vi "BuildGRPCPackages.vi"(11 "CommandLineIn":string[](array[string])) -> (2 "output":string, 3 "return code":i32)   [LabVIEW 2019]
uses:
  <vilib>/JKI/VIPM API/VIPM API_vipm_api.lvlib
panel:
  # "* path to labview sources\n* labview version\n* labview bitness\n* Version"
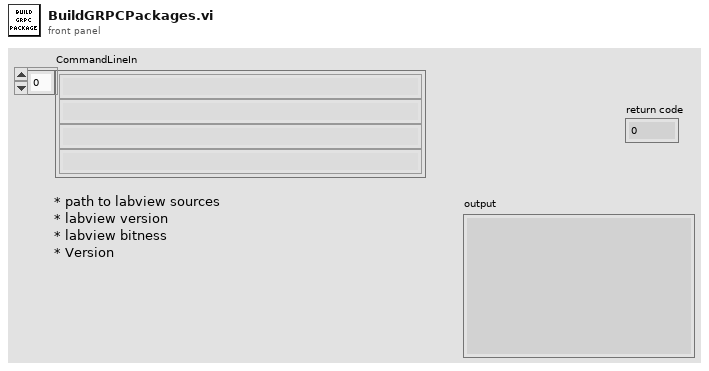
[diagram p1: front panel]
types:
  T1 = typedef "VIPM API_vipm_api.lvlib/LabVIEW Target Info Cluster_vipm_api.ctl" = cluster{"Version":string, "Connection Tested":bool, "Disabled":bool}
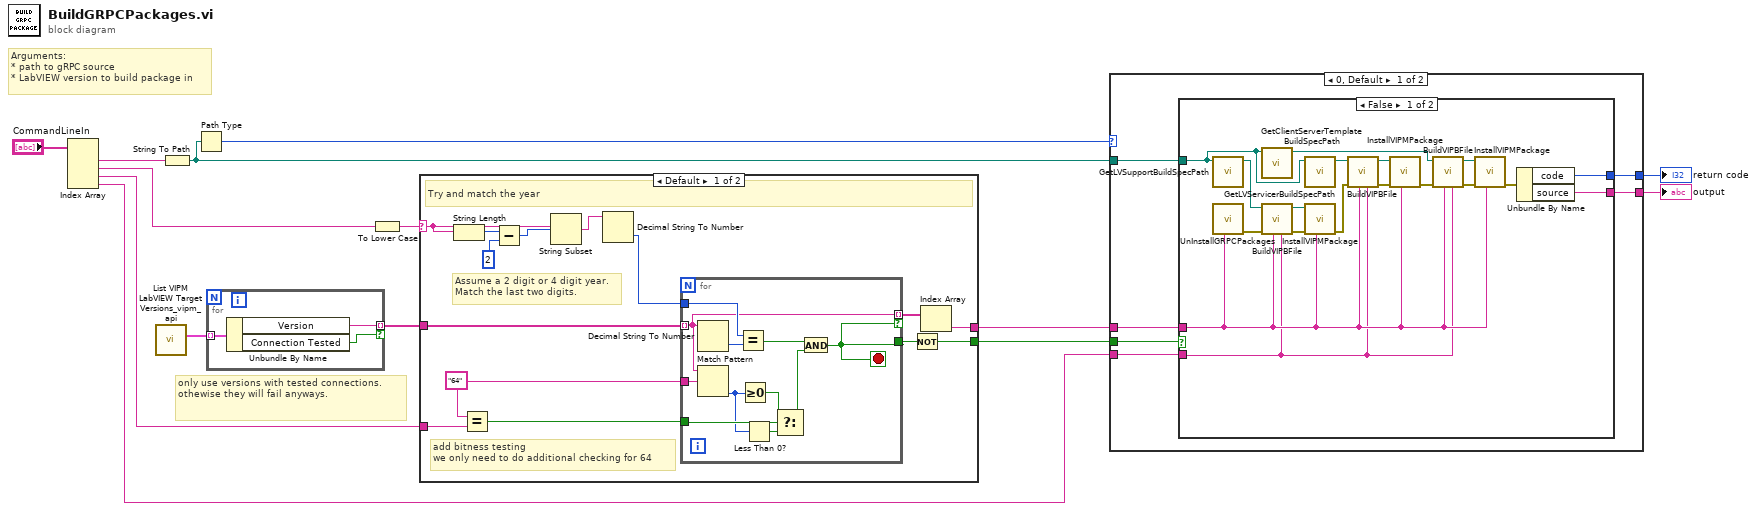
[diagram p0: block diagram]
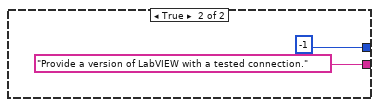
[diagram p2: hidden frame]
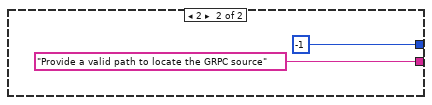
[diagram p3: hidden frame]
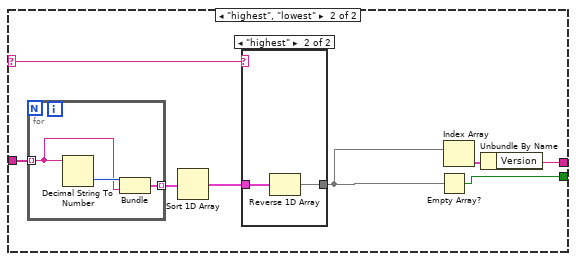
[diagram p4: hidden frame]
diagram:
  # "Arguments:\n* path to gRPC source\n* LabVIEW version to build package in"
  # "only use versions with tested connections.\nothewise they will fail anyways."
  n1 = Index Array(array="CommandLineIn") -> (element #1=w14:string, element #2=w5:string, element #3=w2:string, element #4=w1:string)  [unwired: 4 in]
  n2 = call <vilib>:"List VIPM LabVIEW Target Versions_vipm_api.vi"() -> ("LabVIEW Target Info"=w11:T1[])  [unwired: 10 in, 1 out]
  n3 = String To Path(string=w14) -> (path=w12:path)
  n4 = Path Type(1:w12) -> (0:w13:i16)
  n5 = for {
    tunnel: w11 -> [w17] mode=indexing
    tunnel: [w16] -> w9 mode=indexing if=w15
    n6 = Unbundle By Name(w17) -> ("Version"=w16:string, "Connection Tested"=w15:bool)
  }
  n7 = To Lower Case(string=w5) -> (all lower case string=w10:string)
  n8 = case shown="Default" w10 {
    selector: w10 -> [w31 w48]
    tunnel: w9 -> [w26 w50]
    tunnel: [w22 w45] -> w4
    tunnel: [w21 w43] -> w6
    tunnel: w2 -> [w20 _]
    frame Default {
      w18 = "64" ("x")
      # "add bitness testing\nwe only need to do additional checking for 64"
      # "Assume a 2 digit or 4 digit year.\nMatch the last two digits."
      # "Try and match the year"
      n9 = String Length(string=w31) -> (length=w30:i32)
      n10 = Equal?(x=w18, y=w20) -> (x = y?=w19:bool)
      n11 = Subtract(x=w30, y=2) -> (x-y=w28:i32)
      n12 = String Subset(string=w31, offset (0)=w28) -> (substring=w27:string)  [unwired: 1 in]
      n13 = Decimal String To Number(string=w27) -> (number=w25:i32)  [unwired: 2 in, 1 out]
      n14 = for {
        tunnel: w26 -> [w40] mode=indexing
        tunnel: w25 -> [w41]
        tunnel: [w34] -> w23
        tunnel: [w40] -> w24 mode=indexing if=w34
        tunnel: w19 -> [w37]
        tunnel: w18 -> [w39]
        stop <- w34 stop-if-true
        n15 = Decimal String To Number(string=w40) -> (number=w42:i32)  [unwired: 2 in, 1 out]
        n16 = Match Pattern(string=w40, regular expression=w39) -> (offset past match=w32:i32)  [unwired: 1 in, 3 out]
        n17 = Equal?(x=w41, y=w42) -> (x = y?=w36:bool)
        n18 = Greater Or Equal To 0?(x=w32) -> (x >= 0?=w38:bool)
        n19 = Less Than 0?(x=w32) -> (x < 0?=w33:bool)
        n20 = Select(t=w38, s=w37, f=w33) -> (s? t:f=w35:bool)
        n21 = And(x=w36, y=w35) -> (x .and. y?=w34:bool)
      }
      n22 = Not(x=w23) -> (.not. x?=w21:bool)
      n23 = Index Array(array=w24) -> (element=w22:string)  [unwired: 1 in]
    }
    frame "highest", "lowest" {
      n24 = for {
        tunnel: w50 -> [w55] mode=indexing
        tunnel: [w54] -> w49 mode=indexing
        n25 = Decimal String To Number(string=w55) -> (number=w56:i32)  [unwired: 2 in, 1 out]
        n26 = Bundle(w56, "Version"=w55) -> (w54:cluster{i32, "Version":string})  [unwired: 1 in]
      }
      n27 = Sort 1D Array(array=w49) -> (sorted array=w47:cluster{i32, "Version":string}[])
      n28 = case shown="\"highest\"" w48 {
        tunnel: w47 -> [w51 w53]
        tunnel: [w51 w52] -> w44
        frame Default {
        }
        frame "highest" {
          n29 = Reverse 1D Array(array=w53) -> (reversed array=w52:cluster{i32, "Version":string}[])
        }
      }
      n30 = Empty Array?(array=w44) -> (empty?=w43:bool)
      n31 = Index Array(array=w44) -> (element=w46:cluster{i32, "Version":string})  [unwired: 1 in]
      n32 = Unbundle By Name(w46) -> ("Version"=w45:string)
    }
  }
  n33 = case shown="0, Default" w13 {
    tunnel: [w60 -1 ("return code")] -> w8
    tunnel: [w61 "Provide a valid path to locate the GRPC source" ("Output")] -> w7
    tunnel: w12 -> [w62 _]
    tunnel: w6 -> [w59 _]
    tunnel: w4 -> [w58 _]
    tunnel: w1 -> [w57 _]
    frame 0, Default {
      n34 = case shown="False" w59 {
        tunnel: w62 -> [w78 _]
        tunnel: [w77 "Provide a version of LabVIEW with a tested connection." ("Output")] -> w61
        tunnel: [w76 -1 ("return code")] -> w60
        tunnel: w58 -> [w64 _]
        tunnel: w57 -> [w63 _]
        frame False {
          n35 = call "GetLVSupportBuildSpecPath.vi"("base path"=w78) -> ("build spec path"=w79:path)  [unwired: 10 in]
          n36 = call "UnInstallGRPCPackages.vi"("labview version"=w64) -> ("error out"=w80:errorcluster)  [unwired: 10 in]
          n37 = call "GetClientServerTemplateBuildSpecPath.vi"("base path"=w78) -> ("clientServerTemplateBuildSpecPath"=w68:path)  [unwired: 10 in]
          n38 = call "BuildVIPBFile.vi"("vipb version"=w63, "labview version"=w64, "error in"=w80, "path to vipb file"=w79) -> ("error out"=w74:errorcluster, "build output"=w75:path)  [unwired: 6 in]
          n39 = call "GetLVServicerBuildSpecPath.vi"("base path"=w78) -> ("lv servicer build spec path"=w72:path)  [unwired: 10 in]
          n40 = call "InstallVIPMPackage.vi"("labview version"=w64, "error in"=w74, "vipc file"=w75) -> ("error out"=w73:errorcluster)  [unwired: 8 in]
          n41 = call "BuildVIPBFile.vi"("vipb version"=w63, "labview version"=w64, "error in"=w73, "path to vipb file"=w72) -> ("error out"=w71:errorcluster, "build output"=w70:path)  [unwired: 6 in]
          n42 = call "InstallVIPMPackage.vi"("labview version"=w64, "error in"=w71, "vipc file"=w70) -> ("error out"=w69:errorcluster)  [unwired: 8 in]
          n43 = call "BuildVIPBFile.vi"("vipb version"=w63, "labview version"=w64, "error in"=w69, "path to vipb file"=w68) -> ("error out"=w67:errorcluster, "build output"=w66:path)  [unwired: 6 in]
          n44 = call "InstallVIPMPackage.vi"("labview version"=w64, "error in"=w67, "vipc file"=w66) -> ("error out"=w65:errorcluster)  [unwired: 8 in]
          n45 = Unbundle By Name(w65) -> ("code"=w76:i32, "source"=w77:string)
        }
        frame True {
        }
      }
    }
    frame 2 {
    }
  }
  "return code" <- w8
  "output" <- w7
